vi "Demo_Set_Target_Velocity.vi"() -> ()   [LabVIEW 2016, in "Motor Base.lvlib"]
uses:
  Motor Base.lvclass
  Motor Base.lvlib
panel:
  out "rps":dbl
  in  "stop":bool
  in  "value":dbl=30.0
  in  "Configuration":T1={"Modes of operation"=9, "Feed(pulse)"=1000000, "Max motor speed(r/min)"=12000, "Max torque(0.1%)"=500, "Min position limit(pulse)"=-2147483648, "Max position limit(pulse)"=2147483647} {"Modes of operation" items=["No mode change/no mode assigned"=0, "Profile position mode"=1, "Velocity mode"=2, "Profile velocity mode"=3, "Torque profile mode"=4, "Homing mode"=6, "Interpolated position mode"=7, "Cyclic synchronous position mode"=8, "Cyclic synchronous velocity mode"=9, "Cyclic synchronous torque mode"=10]}
  out "error out":errorcluster
  out "Motor Base out":refnum<class "Motor Base.lvclass">
  in  "error in (no error)":errorcluster
  in  "Connect Info":T2={"Pre_String"="ni.var.io", "Target Name"="PSCM-RT", "Master Name"="EtherCAT Master", "Device Name"="Steering", "PDO Mapping R"="Receive PDO mapping 4", "PDO Mapping T"="Transmit PDO mapping 4"}
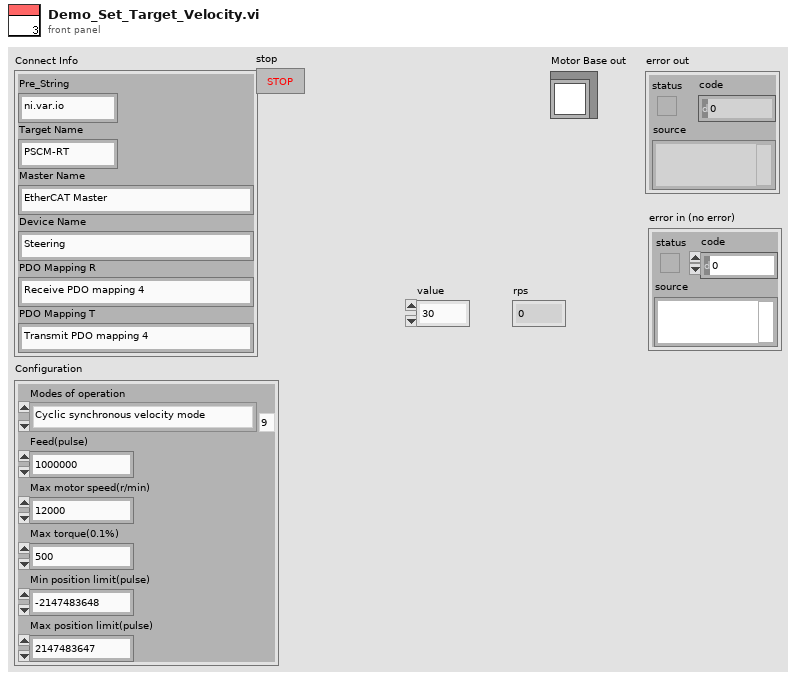
[diagram p1: front panel]
types:
  T1 = cluster{"Modes of operation":i8, "Feed(pulse)":u32, "Max motor speed(r/min)":u32, "Max torque(0.1%)":u16, "Min position limit(pulse)":i32, "Max position limit(pulse)":i32}
  T2 = cluster{"Pre_String":string, "Target Name":string, "Master Name":string, "Device Name":string, "PDO Mapping R":string, "PDO Mapping T":string}
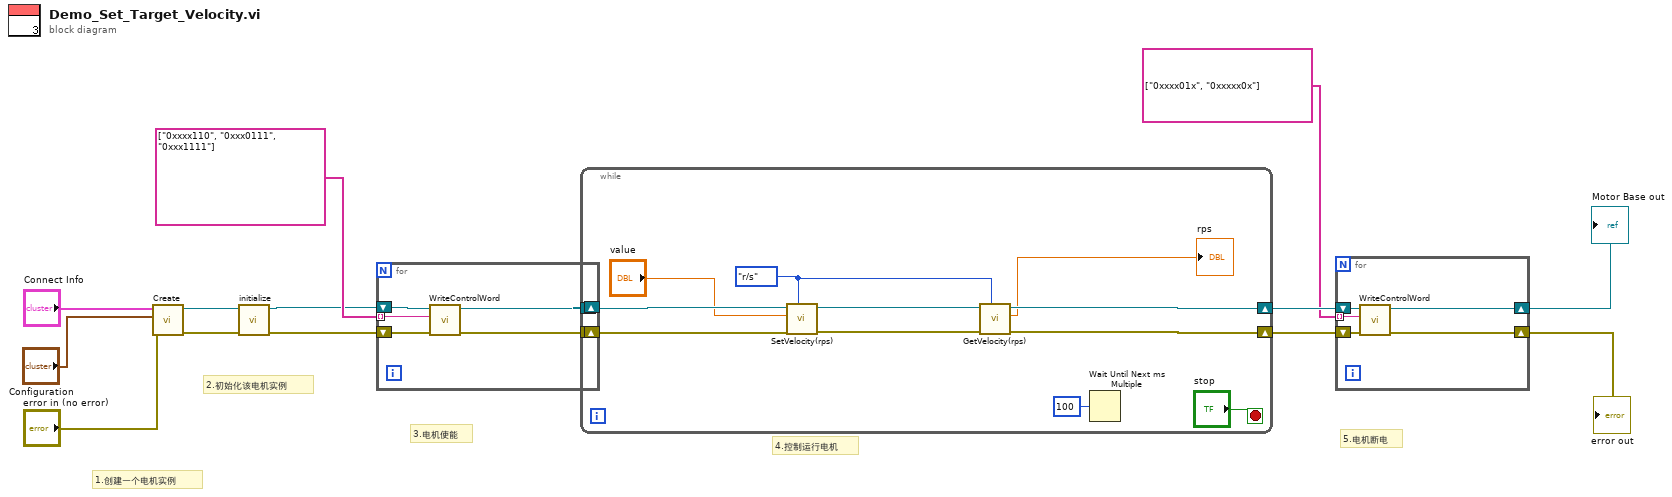
[diagram p0: block diagram]
diagram:
  # "5.电机断电"
  # "4.控制运行电机"
  # "3.电机使能"
  # "2.初始化该电机实例"
  # "1.创建一个电机实例"
  n1 = call "Create.vi"("error in (no error)"="error in (no error)", "Configuration"="Configuration", "Connect Info"="Connect Info") -> ("error out"=w12:errorcluster, "Motor Base out"=w13:refnum<class "Motor Base.lvclass">)  [unwired: 7 in]
  n2 = call-dynamic "initialize.vi"("error in (no error)"=w12, "Motor Base in"=w13) -> ("error out"=w10:errorcluster, "Motor Base out"=w9:refnum<class "Motor Base.lvclass">)  [unwired: 8 in]
  n3 = for {
    tunnel: string[] ["0xxxx110", "0xxx0111", "0xxx1111"] ("ControlWord") -> [w20] mode=indexing
    shift-right: [w18] -> w7
    shift-left: w10 -> [w19]
    shift-right: [w16] -> w8
    shift-left: w9 -> [w17]
    n4 = call-dynamic "WriteControlWord.vi"("error in (no error)"=w19, "Controlword"=w20, "Motor Base in"=w17) -> ("error out"=w18:errorcluster, "Motor Base out"=w16:refnum<class "Motor Base.lvclass">)  [unwired: 7 in]
  }
  n5 = while {
    shift-right: [w29] -> w6
    shift-left: w8 -> [w31]
    shift-right: [w28] -> w5
    shift-left: w7 -> [w30]
    stop <- "stop" stop-if-true
    w21 = enum16{"r/s", "r/m"}."r/s" ("Units")
    n6 = call-dynamic "SetVelocity(rps).vi"("Units"=w21, "error in (no error)"=w30, "velocity"="value", "Motor Base in"=w31) -> ("error out"=w22:errorcluster, "Motor Base out"=w23:refnum<class "Motor Base.lvclass">)  [unwired: 6 in]
    n7 = call-dynamic "GetVelocity(rps).vi"("Units"=w21, "error in (no error)"=w22, "Motor Base in"=w23) -> ("error out"=w28:errorcluster, "rps"=→"rps":dbl, "Motor Base out"=w29:refnum<class "Motor Base.lvclass">)  [unwired: 6 in]
    n8 = Wait Until Next ms Multiple(millisecond multiple=u32 100) -> ()  [unwired: 1 out]
  }
  n9 = for {
    tunnel: string[] ["0xxxx01x", "0xxxxx0x"] ("ControlWord") -> [w36] mode=indexing
    shift-right: [w33] -> w4
    shift-left: w6 -> [w35]
    shift-right: [w32] -> w3
    shift-left: w5 -> [w34]
    n10 = call-dynamic "WriteControlWord.vi"("error in (no error)"=w34, "Controlword"=w36, "Motor Base in"=w35) -> ("error out"=w32:errorcluster, "Motor Base out"=w33:refnum<class "Motor Base.lvclass">)  [unwired: 7 in]
  }
  "Motor Base out" <- w4
  "error out" <- w3
